vi "bundle_unbundle_clusters.vi"() -> ()   [LabVIEW 2026]
panel:
  out "Tank":dbl(slide) scale=0.0..20.0
  out "String":string
  out "Boolean":bool
  out "Numeric":dbl
  in  "Cluster 2":T1
  out "Cluster":T1
  in  "String_ip":string
  in  "Boolean_ip":bool
  in  "Numeric _ip":dbl
  # "CLUSTERS BUNDLE"
  # "CLUSTERS UNBUNDLE"
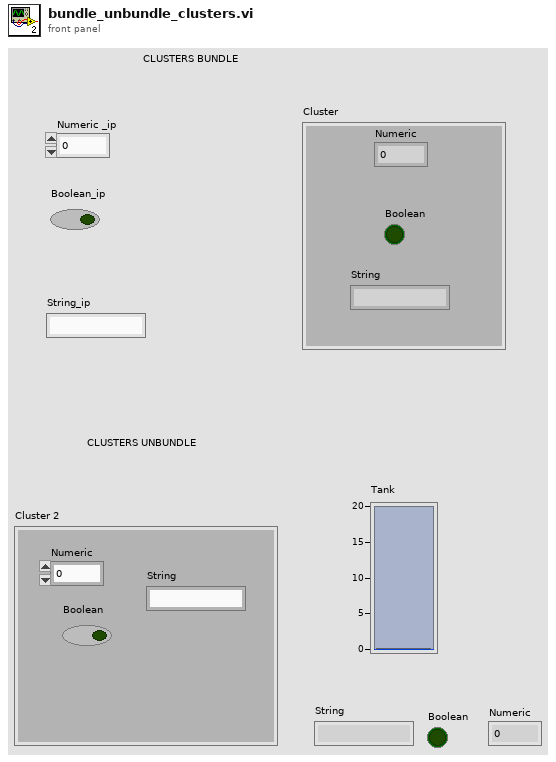
[diagram p1: front panel]
types:
  T1 = cluster{"Numeric":dbl, "Boolean":bool, "String":string}
  T2 = cluster{"Numeric _ip":dbl, "Boolean_ip":bool, "String_ip":string}
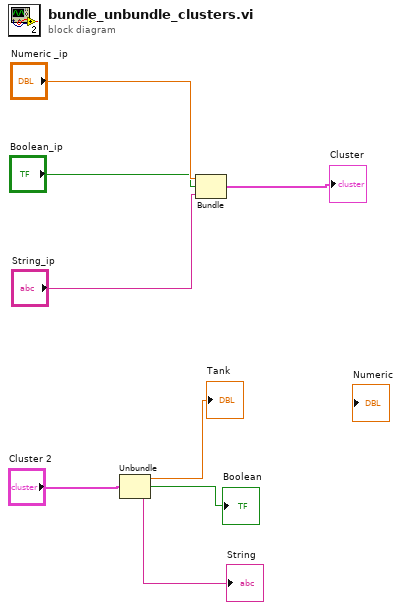
[diagram p0: block diagram]
diagram:
  n1 = Unbundle("Cluster 2") -> ("Numeric"=→"Tank":dbl, "Boolean"=→"Boolean":bool, "String"=→"String":string)
  n2 = Bundle("Numeric _ip"="Numeric _ip", "Boolean_ip"="Boolean_ip", "String_ip"="String_ip") -> (→"Cluster":T2)  [unwired: 1 in]
